vi "Search for IO Support.vi"(7 "Hardware Configuration":T1, 11 "Host Resources":T8) -> (2 "IO supports configuration?":bool)   [LabVIEW 2021, in "Acquisition.lvlib"]
doc: "Search for IO devices in 'Host Resrouces' that support the requested sensors in 'Hardware Configuration'. If sufficient IO is found, then return TRUE for 'IO supports configuration?'"
uses:
  Acquisition.lvlib
  Host Software Package.ctl
  Host IO Resource.ctl
  Host Resources.ctl
  IO Device.ctl
  Channel Settings.ctl
  Interval Timer/Interval Length.ctl
  Interval Timer/Interval Timer.lvlib
  Interval Timer/Repeat Interval.ctl
  Interval Timer/Interval Token.ctl
  IO API.ctl
  Hardware Configuration.ctl
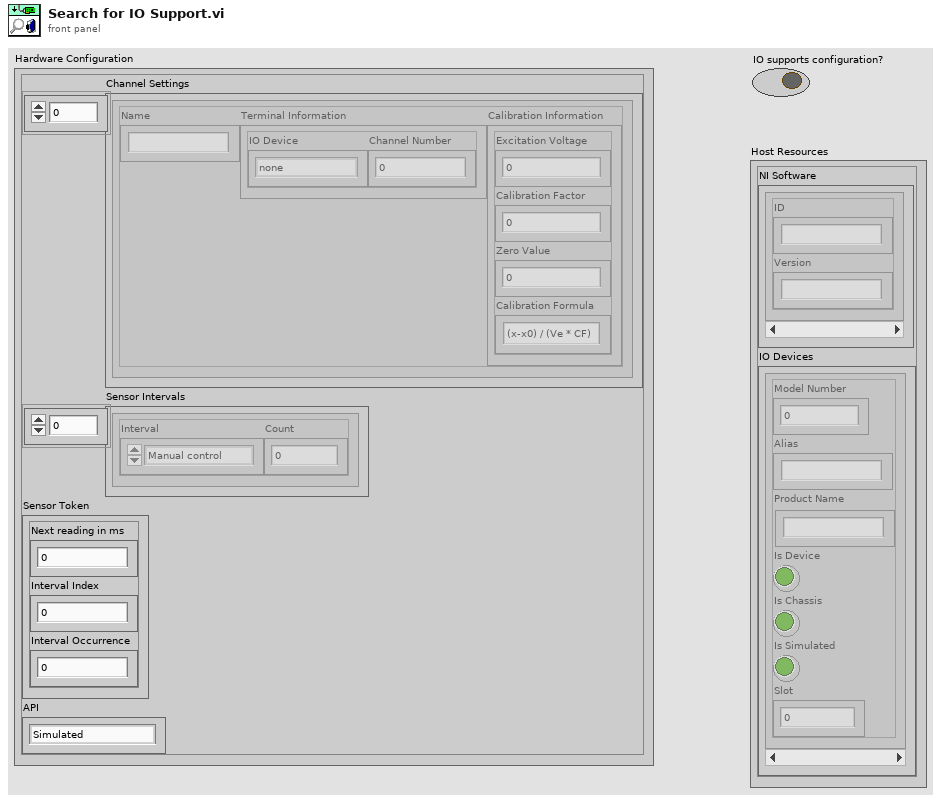
[diagram p1: front panel]
types:
  T1 = typedef "Acquisition.lvlib/Hardware Configuration.ctl" = cluster{"Channel Settings":T2[], "Sensor Intervals":T4[], "Sensor Token":T6, "API":T7}
  T2 = typedef "Acquisition.lvlib/Channel Settings.ctl" = cluster{"Name":string, "Terminal Information":cluster{"IO Device":T3, "Channel Number":i32}, "Calibration Information":cluster{"Excitation Voltage":dbl, "Calibration Factor":dbl, "Zero Value":dbl, "Calibration Formula":string}}
  T3 = typedef "Acquisition.lvlib/IO Device.ctl" = enum16{"none", "9219", "9401"}
  T4 = typedef "Interval Timer.lvlib/Repeat Interval.ctl" = cluster{"Interval":T5, "Count":i32}
  T5 = typedef "Interval Timer.lvlib/Interval Length.ctl" = enum16{"Manual control", "1 second", "10 seconds", "30 seconds", "60 seconds", "600 seconds", "1200 seconds", "3600 seconds"}
  T6 = typedef "Interval Timer.lvlib/Interval Token.ctl" = cluster{"Next reading in ms":u32, "Interval Index":i32, "Interval Occurrence":i32}
  T7 = typedef "Acquisition.lvlib/IO API.ctl" = enum16{"Simulated", "DAQmx"}
  T8 = typedef "Acquisition.lvlib/Host Resources.ctl" = cluster{"NI Software":T9[], "IO Devices":T10[]}
  T9 = typedef "Acquisition.lvlib/Host Software Package.ctl" = cluster{"ID":string, "Version":string}
  T10 = typedef "Acquisition.lvlib/Host IO Resource.ctl" = cluster{"Model Number":u32, "Alias":string, "Product Name":string, "Is Device":bool, "Is Chassis":bool, "Is Simulated":bool, "Slot":i32}
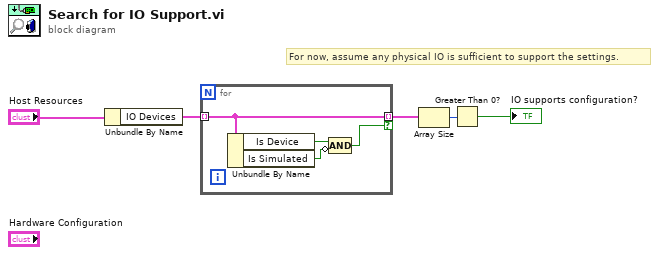
[diagram p0: block diagram]
diagram:
  # "For now, assume any physical IO is sufficient to support the settings."
  n1 = Unbundle By Name("Host Resources") -> ("IO Devices"=w2:T10[])
  n2 = for {
    tunnel: w2 -> [w9] mode=indexing
    tunnel: [w9] -> w3 mode=indexing if=w6
    n3 = Unbundle By Name(w9) -> ("Is Device"=w8:bool, "Is Simulated"=w7:bool)
    n4 = Compound Arithmetic op=AND(w8, invert w7) -> (w6:bool)
  }
  n5 = Array Size(array=w3) -> (size(s)=w4:i32)
  n6 = Greater Than 0?(x=w4) -> (x > 0?=→"IO supports configuration?":bool)
